vi "LSMcontroller_v63_3Dfocus.vi"() -> ()   [LabVIEW 2015] (continued)
                    n4784 = local read "avpp"() -> (w1839:i32)
                    n4785 = local read "Angle ref"() -> (w1838:dbl)
                    n4786 = local read "ROI Type"() -> (w1837:u16)
                    n4787 = local read "xpixels ref"() -> (w1834:i32)
                    n4788 = local read "Vx-min ref"() -> (w1833:dbl)
                    n4789 = local read "Vx-max ref"() -> (w1832:dbl)
                    n4790 = local read "ypixels ref"() -> (w1830:i32)
                    n4791 = local read "Vy-min ref"() -> (w1831:dbl)
                    n4792 = local read "Vy-max ref"() -> (w1827:dbl)
                    n4793 = local read "Sampling rate"() -> (w1821:dbl)
                    n4794 = local read "finite samples"() -> (w1822:bool)
                    n4795 = local read "continuous"() -> (w1825:bool)
                    n4796 = local read "wavdet"() -> (w1826:bool)
                    n4797 = local read "# of frames"() -> (w1824:i32)
                    n4798 = local read "maxbufferAI"() -> (w1823:i32)
                    n4799 = local read "Override AI buffer"() -> (w1819:bool)
                    n4800 = call "2pparameters.vi"("command"="get") -> ("params out"=w1836:T10)  [unwired: 1 in]
                    n4801 = Bundle By Name(cluster=w1836, "type"="X-Y-t movie", "avpp"=w1839, "Angle Img"=w1838, "Xpixels Img"=w1834, "Vx-min Img"=w1833, "VX-max Img"=w1832, "Ypixels Img"=w1830, "Vy-min Img"=w1831, "Vy-max Img"=w1827, "srate"=w1821, "srate Img"=w1821, "finite"=w1822, "cont"=w1825, "wavdet"=w1826, "measpoints"=w1824, "maxbufferAI"=w1823, "Drawing Mode"=w1837, "Vz-reset"=0.0, "AIoverride"=w1819) -> (w1828:T10)
                    n4802 = call "2pparameters.vi"("Params in"=w1828, "command"="set") -> ()  [unwired: 1 out]
                  }
                  frame "X-Y-Z stack" {
                    n4803 = call "2pparameters.vi"("command"="get") -> ("params out"=w1843:T10)  [unwired: 1 in]
                    n4804 = Bundle By Name(cluster=w1843, "type"="X-Y-Z stack") -> (w1841:T10)
                    n4805 = call "2pparameters.vi"("Params in"=w1841, "command"="set") -> ()  [unwired: 1 out]
                  }
                  frame "Lifetime (scan)" {
                    n4806 = call "2pparameters.vi"("command"="get") -> ("params out"=w1848:T10)  [unwired: 1 in]
                    n4807 = Bundle By Name(cluster=w1848, "type"="Lifetime (scan)") -> (w1846:T10)
                    n4808 = call "2pparameters.vi"("Params in"=w1846, "command"="set") -> ()  [unwired: 1 out]
                  }
                  frame "Lifetime (contour)" {
                    n4809 = local read "Vy-min draw"() -> (w1858:dbl)
                    n4810 = local read "Vy-max draw"() -> (w1857:dbl)
                    n4811 = local read "Vx-min draw"() -> (w1860:dbl)
                    n4812 = local read "Vx-max draw"() -> (w1859:dbl)
                    n4813 = local read "xpixels ref"() -> (w1856:i32)
                    n4814 = local read "ypixels ref"() -> (w1855:i32)
                    n4815 = local read "ROI Type"() -> (w1854:u16)
                    n4816 = local read "srateAODOtt"() -> (w1865:dbl)
                    n4817 = local read "# of frames"() -> (w1870:i32)
                    n4818 = local read "refreshtime"() -> (w1862:dbl)
                    n4819 = local read "Pel"() -> (w1853:dbl)
                    n4820 = local read "bin"() -> (w1868:dbl)
                    n4821 = local read "Override AI buffer"() -> (w1851:bool)
                    n4822 = local read "finite samples"() -> (w1877:bool)
                    n4823 = local read "srateAODOtt"() -> (w1864:dbl)
                    n4824 = local read "srateAODOtt"() -> (w1871:dbl)
                    n4825 = local read "continuous"() -> (w1876:bool)
                    n4826 = local read "Angle ref"() -> (w1861:dbl)
                    n4827 = local read "wavdet"() -> (w1878:bool)
                    n4828 = local read "Vx-ref"() -> (w1873:dbl)
                    n4829 = local read "Vy-ref"() -> (w1875:dbl)
                    n4830 = local read "avpp"() -> (w1874:i32)
                    n4831 = call "tt_timeandsamples.vi"("bin"=w1868, "refreshtime"=w1862, "srateAODOtt"=w1865, "tot#ofsamples"=w1870) -> ("refreshrate"=w1866:dbl, "refreshbuffer"=w1867:i32, "timetracecycles"=w1872:i32)  [unwired: 5 in]
                    n4832 = local read "bin"() -> (w1869:dbl)
                    n4833 = call "2pparameters.vi"("command"="get") -> ("params out"=w1881:T10)  [unwired: 1 in]
                    n4834 = Bundle By Name(cluster=w1881, "Drawing Mode"=w1854, "measpoints"=w1870, "tt_cycles"=w1872, "refreshbuffer"=w1867, "refreshrate"=w1866, "Vx-ref"=w1873, "Vy-ref"=w1875, "srate"=w1864, "finite"=w1877, "cont"=w1876, "wavdet"=w1878, "avpp"=w1874, "srateAODO"=w1871, "bufferAI"=w1867, "bin"=w1869, "Angle Img"=w1861, "Vxminref"=w1860, "Vxmaxref"=w1859, "Vyminref"=w1858, "Vymaxref"=w1857, "Xpixels Img"=w1856, "Ypixels Img"=w1855, "Pel"=w1853, "Vz-reset"=0.0, "AIoverride"=w1851, "type"="Lifetime (contour)") -> (w1879:T10)
                    n4835 = Reciprocal(x=w1866) -> (1/x=w1863:dbl)
                    n4836 = local write "refreshtime"(w1863) -> ()
                    n4837 = call "2pparameters.vi"("Params in"=w1879, "command"="set") -> ()  [unwired: 1 out]
                  }
                  frame "X-Y-Z-t movie" {
                  }
                  frame "linescan" {
                  }
                  frame "Timetrace" {
                    n4838 = local read "Vy-min draw"() -> (w1891:dbl)
                    n4839 = local read "Vy-max draw"() -> (w1890:dbl)
                    n4840 = local read "Vx-min draw"() -> (w1893:dbl)
                    n4841 = local read "Vx-max draw"() -> (w1892:dbl)
                    n4842 = local read "xpixels ref"() -> (w1889:i32)
                    n4843 = local read "ypixels ref"() -> (w1888:i32)
                    n4844 = local read "ROI Type"() -> (w1887:u16)
                    n4845 = local read "srateAODOtt"() -> (w1898:dbl)
                    n4846 = local read "# of frames"() -> (w1903:i32)
                    n4847 = local read "refreshtime"() -> (w1895:dbl)
                    n4848 = local read "Pel"() -> (w1886:dbl)
                    n4849 = local read "bin"() -> (w1901:dbl)
                    n4850 = local read "Override AI buffer"() -> (w1884:bool)
                    n4851 = local read "finite samples"() -> (w1910:bool)
                    n4852 = local read "srateAODOtt"() -> (w1897:dbl)
                    n4853 = local read "srateAODOtt"() -> (w1904:dbl)
                    n4854 = local read "continuous"() -> (w1909:bool)
                    n4855 = local read "Angle ref"() -> (w1894:dbl)
                    n4856 = local read "wavdet"() -> (w1911:bool)
                    n4857 = local read "Vx-ref"() -> (w1906:dbl)
                    n4858 = local read "Vy-ref"() -> (w1908:dbl)
                    n4859 = local read "avpp"() -> (w1907:i32)
                    n4860 = call "tt_timeandsamples.vi"("bin"=w1901, "refreshtime"=w1895, "srateAODOtt"=w1898, "tot#ofsamples"=w1903) -> ("refreshrate"=w1899:dbl, "refreshbuffer"=w1900:i32, "timetracecycles"=w1905:i32)  [unwired: 5 in]
                    n4861 = local read "bin"() -> (w1902:dbl)
                    n4862 = call "2pparameters.vi"("command"="get") -> ("params out"=w1914:T10)  [unwired: 1 in]
                    n4863 = Bundle By Name(cluster=w1914, "Drawing Mode"=w1887, "measpoints"=w1903, "tt_cycles"=w1905, "refreshbuffer"=w1900, "refreshrate"=w1899, "Vx-ref"=w1906, "Vy-ref"=w1908, "srate"=w1897, "finite"=w1910, "cont"=w1909, "wavdet"=w1911, "avpp"=w1907, "srateAODO"=w1904, "bufferAI"=w1900, "bin"=w1902, "Angle Img"=w1894, "Vxminref"=w1893, "Vxmaxref"=w1892, "Vyminref"=w1891, "Vymaxref"=w1890, "Xpixels Img"=w1889, "Ypixels Img"=w1888, "Pel"=w1886, "Vz-reset"=0.0, "AIoverride"=w1884, "type"="Timetrace") -> (w1912:T10)
                    n4864 = Reciprocal(x=w1899) -> (1/x=w1896:dbl)
                    n4865 = local write "refreshtime"(w1896) -> ()
                    n4866 = call "2pparameters.vi"("Params in"=w1912, "command"="set") -> ()  [unwired: 1 out]
                  }
                  frame "Lifetime (point)" {
                  }
                }
              }
              frame #1 {
                w1917 = FALSE ("wavdet")
                n4867 = call "2pparameters.vi"("command"="get") -> ("params out"=w1921:T10)  [unwired: 1 in]
                n4868 = Bundle By Name(cluster=w1921, "finite"=w1917, "cont"=w1917, "wavdet"=TRUE) -> (w1918:T10)
                n4869 = call "2pparameters.vi"("Params in"=w1918, "command"="set") -> ()  [unwired: 1 out]
              }
              frame #2 {
                n4870 = property on="Loaded settings" class="Ring (strict)"() -> ("RingText.Text"=w1923:string)  [unwired: 2 in, 2 out]
                n4871 = control-ref of="Analog Lines Plot"() -> (w1925:refnum<vi>)
                n4872 = control-ref of="Digital Lines Plot"() -> (w1924:refnum<vi>)
                n4873 = call "Usedlinesfromsettingsfile.vi"("sertting"=w1923) -> ("used AO names"=w1929:string[], "used AO lines"=w1928:tag[], "used DO names"=w1927:string[], "used DO lines"=w1926:tag[])
                n4874 = call "loadAODOwfparamsfromsettingsfile.vi"("sertting"=w1923) -> ()
                n4875 = call "prepAOWaveplot.vi"("WaveformGraph in"=w1925, "Analog Used Names"=w1929) -> ()  [unwired: 1 in]
                n4876 = local write "Analog Used Names"(w1929) -> ()
                n4877 = local write "Analog Used Lines"(w1928) -> ()
                n4878 = call "prepDOWaveplot.vi"("DigitalGraph in"=w1924, "used DO names"=w1927) -> ()  [unwired: 1 in]
                n4879 = local write "Digital Used Names"(w1927) -> ()
                n4880 = local write "Digital Used Lines"(w1926) -> ()
              }
              frame #3 {
                n4881 = call "waveformparamsv2.vi"("command"="get") -> ("Params out"=w1946:T14)  [unwired: 4 in, 2 out]
                n4882 = Unbundle By Name(w1946) -> ("AO parameters"=w1947:T15, "DO parameters"=w1948:T17)
                n4883 = for {
                  tunnel: w1947 -> [w1967] mode=indexing
                  tunnel: [w1965] -> w1949 mode=indexing
                  tunnel: [w1964] -> w1934 mode=indexing
                  tunnel: [w1962] -> w1937 mode=indexing
                  i -> [w1966]
                  n4884 = Unbundle By Name(w1967) -> ("AOtab"=w1968:dbl)
                  n4885 = case shown="0, Default" w1968 {
                    tunnel: w1967 -> [_ w1979 w1981 w1983]
                    tunnel: [_ w1978 w1980 w1982] -> w1963
                    frame -1 {
                    }
                    frame 0, Default {
                      n4886 = call "generateRampedSquareWave_fromAOparameters.vi"("AO params"=w1979) -> ("Waveform"=w1978:waveform(dbl))  [unwired: 1 out]
                    }
                    frame 1 {
                      n4887 = call "generateTriWave_fromAOparameters.vi"("AO params"=w1981) -> ("Waveform"=w1980:waveform(dbl))  [unwired: 1 out]
                    }
                    frame 2 {
                      n4888 = call "matlabAOwffromparam.vi"("Cluster"=w1983) -> ("Waveform"=w1982:waveform(dbl))  [unwired: 1 out]
                    }
                  }
                  n4889 = case shown="0" w1966 {
                    tunnel: [w1973 -1] -> w1965
                    tunnel: [w1972 w1976] -> w1964
                    tunnel: w1963 -> [w1972 w1976]
                    tunnel: [w1969 -1.0] -> w1962
                    frame 0 {
                      n4890 = Unbundle By Name(w1972) -> ("dt"=w1971:dbl, "Y"=w1974:dbl[])
                      n4891 = Reciprocal(x=w1971) -> (1/x=w1970:dbl)
                      n4892 = Array Size(array=w1974) -> (size(s)=w1973:i32)
                      n4893 = Round To Nearest(number=w1970) -> (nearest integer value=w1969:dbl)
                    }
                    frame 1, Default {
                    }
                  }
                }
                n4894 = Index Array(array=w1949, index=0) -> (element=w1951:i32)
                n4895 = Index Array(array=w1937, index=0) -> (element=w1936:dbl)
                n4896 = for {
                  tunnel: w1948 -> [w1956] mode=indexing
                  tunnel: [w1954] -> w1935 mode=indexing
                  tunnel: w1951 -> [w1953]
                  n4897 = Unbundle By Name(w1956) -> ("DOtab"=w1955:dbl)
                  n4898 = case shown="0, Default" w1955 {
                    tunnel: w1956 -> [w1959 w1961]
                    tunnel: w1953 -> [w1958 _]
                    tunnel: [w1957 w1960] -> w1954
                    frame 0, Default {
                      n4899 = call "simple digital from wf params.vi"("waveform params"=w1959, "number of samples"=w1958) -> ("digital waveform"=w1957:digitalwaveform)
                    }
                    frame 1 {
                      n4900 = call "matlabDOwffromparam.vi"("waveform params"=w1961) -> ("digital waveform"=w1960:digitalwaveform)
                    }
                  }
                }
                n4901 = property on="refwf" class="Ring (strict)"() -> ("RingText.Text"=w1939:string)  [unwired: 2 in, 2 out]
                n4902 = call "correctwaveformsizetemp.vi"("new sampling frequency (Hz)"=w1936, "start"=FALSE, "reference waveforms to"=w1939, "Analog waveforms in"=w1934, "stop"=FALSE, "Digital waveforms in"=w1935) -> ("analog wf out"=w1933:waveform(dbl)[], "Digital wf out"=w1932:digitalwaveform[], "measpoints"=w1930:i32)
                n4903 = local read "wavdet"() -> (w1931:bool)
                n4904 = case shown="True" w1931 {
                  tunnel: w1930 -> [_ w1952]
                  frame False {
                  }
                  frame True {
                    n4905 = local write "# of frames"(w1952) -> ()
                  }
                }
                n4906 = local write "Analog Lines Plot"(w1933) -> ()
                n4907 = local write "Digital Lines Plot"(w1932) -> ()
                n4908 = call "GetNumCamFramesv2.vi"("Digital Waveform Graph"=w1932) -> ("Numeric"=w1944:i32)  [unwired: 10 in]
                n4909 = call "waveformsAObuffer.vi"("AO wf in"=w1933, "command"="set") -> ()  [unwired: 1 out]
                n4910 = call "waveformsDObuffer.vi"("DO wf in"=w1932, "command"="set") -> ()  [unwired: 1 out]
                n4911 = local write "Total Camera Frames"(w1944) -> ()
              }
              frame #4 {
                n4912 = local read "AO channels"() -> (w1984:u32)
                n4913 = call "2pparameters.vi"("command"="get") -> ("params out"=w1986:T10)  [unwired: 1 in]
                n4914 = Unbundle By Name(w1986) -> ("aAO"=w1985:u32[])
                n4915 = Search 1D Array(1D array=w1985, element=w1984) -> (index of element=w1988:i32)  [unwired: 1 in]
                n4916 = Equal?(x=w1988, y=-1.0) -> (x = y?=w1989:bool)
                n4917 = case shown="False" w1989 {
                  tunnel: w1988 -> [w2014 _]
                  frame False {
                    n4918 = call "waveformparamsv2.vi"("command"="get") -> ("Params out"=w1997:T14)  [unwired: 4 in, 2 out]
                    n4919 = Unbundle By Name(w1997) -> ("AO parameters"=w1996:T15)
                    n4920 = Index Array(array=w1996, index=w2014) -> (element=w2013:T16)
                    n4921 = Unbundle By Name(w2013) -> ("AOtab"=w1994:dbl, "Repeats"=w2012:dbl, "Cycles"=w2011:dbl, "Start amplitude (V)"=w2010:dbl, "Baseline (V)"=w2009:dbl, "Step size (V)"=w2008:dbl, "DC (%)"=w2007:dbl, "Sampling frequency (Hz)"=w2006:dbl, "Period (ms)"=w2005:dbl, "Offset (V)"=w2004:dbl, "Amplitude (V)"=w2003:dbl, "Frequency"=w2002:dbl, "Tri Repeats"=w2001:dbl, "phase shift (ms)"=w2000:dbl, "Pulses"=w1999:dbl, "Tri phase"=w1995:dbl, "padding value"=w1991:dbl, "Matlab wave file"=w1992:path)
                    n4922 = To Unsigned Long Integer(number=w1994) -> (unsigned 32bit integer=w1993:u32)
                    n4923 = local write "Build analog waveform tabs"(w1993) -> ()
                    n4924 = local write "Matlab waveform path"(w1992) -> ()
                    n4925 = local write "phase shift (ms)"(w2000) -> ()
                    n4926 = local write "Repeats"(w2012) -> ()
                    n4927 = local write "Cycles"(w2011) -> ()
                    n4928 = local write "Amplitude (V)"(w2003) -> ()
                    n4929 = local write "Matlab padding value"(w1991) -> ()
                    n4930 = local write "Tri padding value"(w1991) -> ()
                    n4931 = local write "Start amplitude (V)"(w2010) -> ()
                    n4932 = local write "Tri Phase (s)"(w1995) -> ()
                    n4933 = local write "Period (ms)"(w2005) -> ()
                    n4934 = local write "Tri Repeats"(w2001) -> ()
                    n4935 = local write "Offset (V)"(w2004) -> ()
                    n4936 = local write "Frequency"(w2002) -> ()
                    n4937 = local write "Pulses"(w1999) -> ()
                    n4938 = local write "padding value"(w1991) -> ()
                    n4939 = local write "Sampling rate \ncurrent wf"(w2006) -> ()
                    n4940 = local write "Baseline (V)"(w2009) -> ()
                    n4941 = local write "Step size (V)"(w2008) -> ()
                    n4942 = local write "DC (%)"(w2007) -> ()
                  }
                  frame True {
                  }
                }
              }
              frame #5 {
                n4943 = local read "DO channels"() -> (w2017:u16)
                n4944 = call "2pparameters.vi"("command"="get") -> ("params out"=w2019:T10)  [unwired: 1 in]
                n4945 = Unbundle By Name(w2019) -> ("aDO"=w2018:u32[])
                n4946 = Search 1D Array(1D array=w2018, element=w2017) -> (index of element=w2016:i32)  [unwired: 1 in]
                n4947 = Equal?(x=w2016, y=-1.0) -> (x = y?=w2015:bool)
                n4948 = case shown="False" w2015 {
                  tunnel: w2016 -> [w2034 _]
                  frame False {
                    n4949 = call "waveformparamsv2.vi"("command"="get") -> ("Params out"=w2028:T14)  [unwired: 4 in, 2 out]
                    n4950 = Unbundle By Name(w2028) -> ("DO parameters"=w2026:T17)
                    n4951 = Index Array(array=w2026, index=w2034) -> (element=w2033:T18)
                    n4952 = Unbundle By Name(w2033) -> ("Digital DC (%)"=w2032:dbl, "Digital phase"=w2031:dbl, "Digital Freq (Hz)"=w2030:dbl, "Sampling frequency (Hz)"=w2029:dbl, "Digital time offset (s)"=w2025:dbl, "padding value"=w2024:dbl, "matlab wave file"=w2023:path, "DOtab"=w2022:dbl)
                    n4953 = local write "Build digital waveform tabs"(w2022) -> ()
                    n4954 = local write "Digital DC (%)"(w2032) -> ()
                    n4955 = local write "Matlab waveform path DO"(w2023) -> ()
                    n4956 = local write "Sampling rate \ncurrent wf"(w2029) -> ()
                    n4957 = local write "Digital time offset (s)"(w2025) -> ()
                    n4958 = local write "Matlab padding value DO"(w2024) -> ()
                    n4959 = local write "Digital padding value"(w2024) -> ()
                    n4960 = local write "Digital Freq (Hz)"(w2030) -> ()
                    n4961 = local write "Digital phase (s)"(w2031) -> ()
                  }
                  frame True {
                  }
                }
              }
              frame #6 {
                n4962 = local read "finite samples"() -> (w2035:bool)
                n4963 = local read "continuous"() -> (w2036:bool)
                n4964 = local read "wavdet"() -> (w2037:bool)
                n4965 = call "2pparameters.vi"("command"="get") -> ("params out"=w2040:T10)  [unwired: 1 in]
                n4966 = Bundle By Name(cluster=w2040, "finite"=w2035, "cont"=w2036, "wavdet"=w2037) -> (w2038:T10)
                n4967 = call "2pparameters.vi"("Params in"=w2038, "command"="set") -> ()  [unwired: 1 out]
              }
            }
          }
          event "Exit": Value Change {
            n4968 = event-data() -> ("NewVal"=w2042:bool)  [unwired: 1 in]
          }
        }
        n4969 = Wait (ms)(milliseconds to wait=u32 50) -> ()  [unwired: 1 out]
      }
    }
    frame #3 {
      w6446 = FALSE ("Value (Signaling)")
      n4970 = property on="Start" class="Bool (strict)"("Val(Sgnl)"=w6446) -> ()  [unwired: 2 in, 2 out]
      n4971 = property on="Exit" class="Bool (strict)"("Val(Sgnl)"=w6446) -> ()  [unwired: 2 in, 2 out]
      n4972 = property on="Stop" class="Bool (strict)"("Val(Sgnl)"=w6446) -> ()  [unwired: 2 in, 2 out]
      n4973 = flat-sequence {
        frame #0 {
          w6447 = u16 1 items=["OD 0"=1, "OD 0.5"=2, "OD 1"=3, "OD 2"=4, "OD 3"=5, "OD 4"=6] ("New ODfilt")
          n4974 = local read "ODfilt"() -> (w6448:u16)
          n4975 = call "filterwheelcontrol_nothorlabslib.vi"("Current OD filt"=w6448, "New ODfilt"=w6447) -> ()  [unwired: 1 in]
        }
        frame #1 {
          n4976 = Wait (ms)(milliseconds to wait=u32 1000) -> ()  [unwired: 1 out]
        }
      }
    }
  }
